vi "IMAQdx Enumerate Attributes.vi"(5 "Visibility":T1=enum."Advanced", 7 "Root":string, 8 "error in":errorcluster, 11 "Session In":T2) -> (0 "error out":errorcluster, 2 "Attribute Information Array":T4(array[cluster]), 3 "Session Out":T2)   [LabVIEW 2013, in "NI_Vision_Acquisition_Software.lvlib"]
doc: "Gets the attributes supported by the camera."
uses:
  NI_Vision_Acquisition_Software.lvlib
  IMAQdx Attribute Type.ctl
  IMAQdx.ctl
  IMAQdx Attribute Visibility.ctl
  niimaqdx.dll
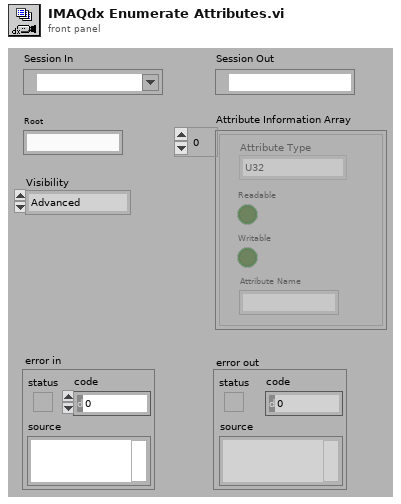
[diagram p1: front panel]
types:
  T1 = typedef "NI_Vision_Acquisition_Software.lvlib/IMAQdx Attribute Visibility.ctl" = enum32{"Simple", "Intermediate", "Advanced"}
  T2 = typedef "IMAQdx.ctl" = refnum<k21>
  T3 = typedef "NI_Vision_Acquisition_Software.lvlib/IMAQdx Attribute Type.ctl" = enum32{"U32", "I64", "DBL", "String", "Enum", "Bool", "Command"}
  T4 = cluster{"Attribute Type":T3, "Readable":bool, "Writable":bool, "Attribute Name":string}[]
  T5 = cluster{"Attribute Type":u32, "Readable":bool, "Writeable":bool, "Attribute Name":string}[]
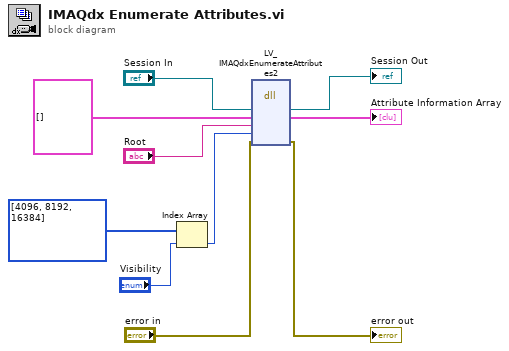
[diagram p0: block diagram]
diagram:
  n1 = Index Array(array=u32[] [4096, 8192, 16384], index="Visibility") -> (element=w1:u32)
  n2 = dll-call lib="niimaqdx.dll" fn="LV_IMAQdxEnumerateAttributes2"("Session In"="Session In", "Attribute Information Array"=T5 [], "attributeRoot"="Root", "visibility"=w1, "error in"="error in") -> ("Session In"=→"Session Out":T2, "Attribute Information Array"=→"Attribute Information Array":T5, "error in"=→"error out":errorcluster)  [unwired: 6 in, 2 out]
